vi "Parse Diff Report to Text.vi"(0 "XML Path":path, 1 "Ignore cosmetic changes? (T)":bool=TRUE, 2 "Attributes only? (F)":bool, 11 "error in":errorcluster) -> (4 "change description":string, 15 "error out":errorcluster)   [LabVIEW 2020, in "Graphical Diff.lvlib"]
uses:
  Graphical Diff.lvlib
  <vilib>/xml/NI_XML.lvlib
  <resource>/objmgr/DOMUserDefRef.rc
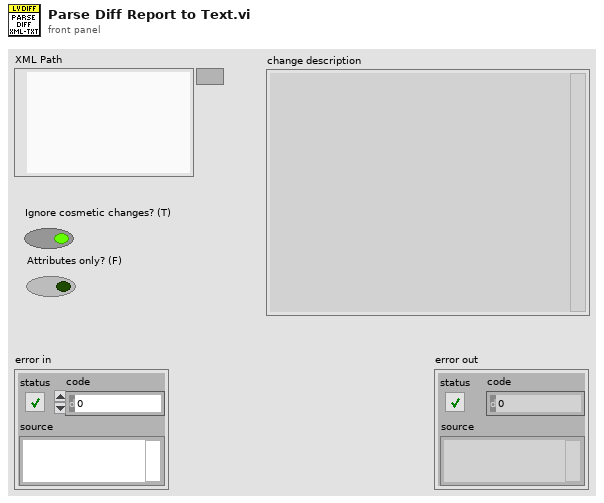
[diagram p1: front panel]
types:
  T1 = cluster{"Value":string, "Value":string, "Value":string, "Value":string}
  T2 = cluster{"Value":string, "Value":string, "Value":string, "Value":string}[]
  T3 = cluster{string, cluster{"Value":string, "Value":string, "Value":string, "Value":string}[]}
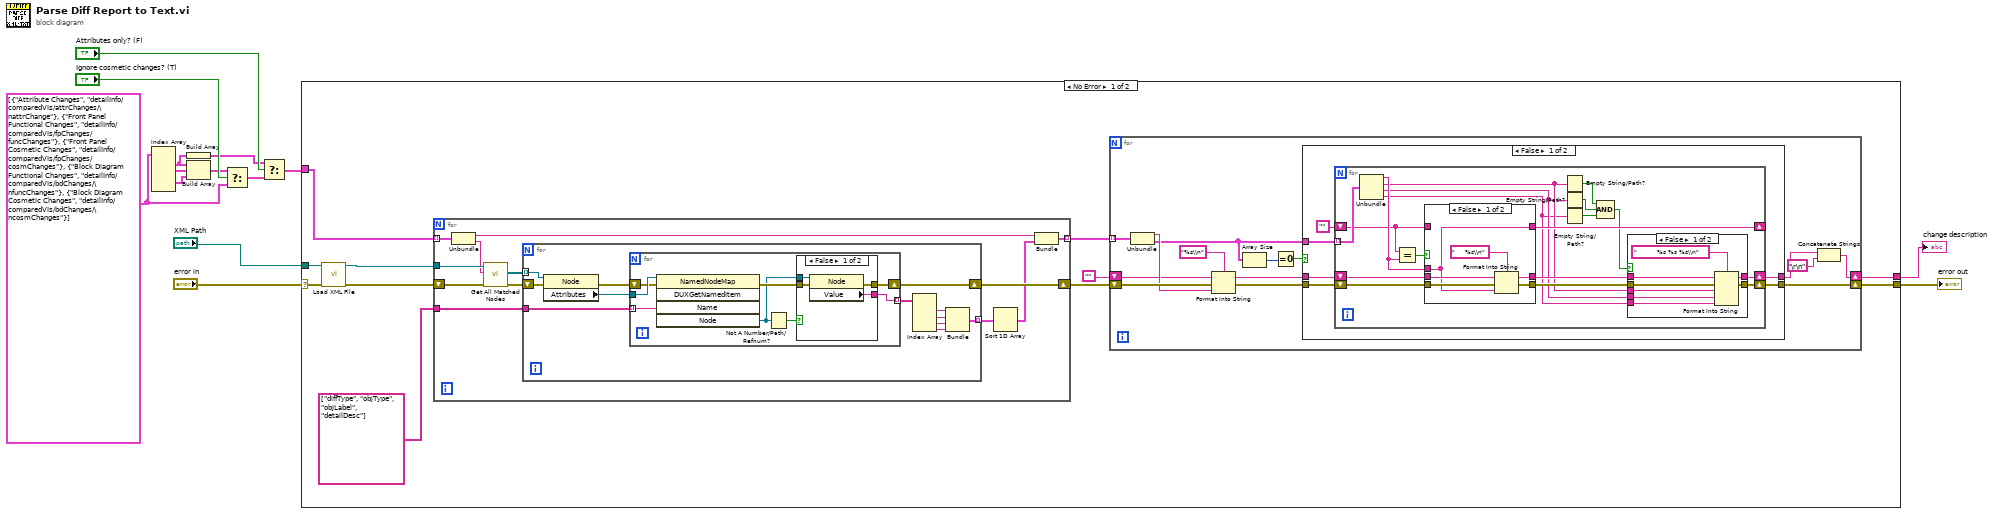
[diagram p0: block diagram]
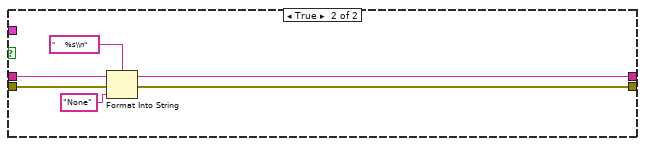
[diagram p4: hidden frame]
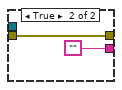
[diagram p5: hidden frame]
diagram:
  w5 = cluster{string, string}[] [{"Attribute Changes", "detailInfo/comparedVIs/attrChanges/\nattrChange"}, {"Front Panel Functional Changes", "detailInfo/comparedVIs/fpChanges/funcChanges"}, {"Front Panel Cosmetic Changes", "detailInfo/comparedVIs/fpChanges/cosmChanges"}, {"Block Diagram Functional Changes", "detailInfo/comparedVIs/bdChanges/\nfuncChanges"}, {"Block Diagram Cosmetic Changes", "detailInfo/comparedVIs/bdChanges/\ncosmChanges"}]
  n1 = Index Array(array=w5) -> (element #1=w8:cluster{string, string}, element #2=w9:cluster{string, string}, element #4=w10:cluster{string, string})  [unwired: 5 in, 2 out]
  n2 = Build Array(w8) -> (w3:cluster{string, string}[])
  n3 = Build Array(w8, w9, w10) -> (w6:cluster{string, string}[])
  n4 = Select(t=w6, s="Ignore cosmetic changes? (T)", f=w5) -> (s? t:f=w1:cluster{string, string}[])
  n5 = Select(t=w3, s="Attributes only? (F)", f=w1) -> (s? t:f=w2:cluster{string, string}[])
  n6 = case shown="No Error" "error in" {
    selector: "error in" -> [w25 w127]
    tunnel: "XML Path" -> [w24 _]
    tunnel: [w22 w127] -> w12
    tunnel: [w21 _] -> w11
    tunnel: w2 -> [w15 _]
    frame No Error {
      n7 = call <vilib>:"Load XML File.vi"("path to XML document"=w24, "error in (no error)"=w25) -> ("DOM document out"=w20:refnum<k20>, "error out"=w19:errorcluster)  [unwired: 11 in, 1 out]
      n8 = for {
        tunnel: w20 -> [w100]
        shift-right: [w97] -> w16
        shift-left: w19 -> [w99]
        tunnel: w15 -> [w94] mode=indexing
        tunnel: string[] ["diffType", "objType", "objLabel", "detailDesc"] -> [w96]
        tunnel: [w89] -> w18 mode=indexing
        n9 = Unbundle(w94) -> (w90:string, w93:string)
        n10 = call <vilib>:"Get All Matched Nodes.vi"("error in (no error)"=w99, "XPath expression"=w93, "node in"=w100) -> ("error out"=w98:errorcluster, "node result array"=w92:refnum<k20>[])  [unwired: 6 in, 1 out]
        n11 = for {
          shift-right: [w109] -> w97
          shift-left: w98 -> [w110]
          tunnel: w96 -> [w108]
          tunnel: [w102] -> w95 mode=indexing
          tunnel: w92 -> [w101] mode=indexing
          n12 = property class="Node"(reference=w101, error in=w110) -> (error out=w112:errorcluster, "Attributes"=w111:refnum<k20>)  [unwired: 1 out]
          n13 = for {
            tunnel: w111 -> [w120]
            shift-right: [w116] -> w109
            shift-left: w112 -> [w119]
            tunnel: w108 -> [w118] mode=indexing
            tunnel: [w115] -> w107 mode=indexing
            n14 = invoke class="NamedNodeMap" method="DUXGetNamedItem"(reference=w120, error in=w119, "Name"=w118) -> (error out=w117:errorcluster, "Node"=w113:refnum<k20>)  [unwired: 2 in, 3 out]
            n15 = Not A Number/Path/Refnum?(number/path/refnum=w113) -> (NaN/Path/Refnum?=w114:bool)
            n16 = case shown="False" w114 {
              tunnel: w117 -> [w124 w126]
              tunnel: [w123 w126] -> w116
              tunnel: [w122 ""] -> w115
              tunnel: w113 -> [w121 _]
              frame False {
                n17 = property class="Node"(reference=w121, error in=w124) -> (error out=w123:errorcluster, "Value"=w122:string)  [unwired: 1 out]
              }
              frame True {
              }
            }
          }
          n18 = Index Array(array=w107) -> (element #1=w103:string, element #2=w106:string, element #3=w104:string, element #4=w105:string)  [unwired: 4 in]
          n19 = Bundle("Value"=w103, "Value"=w106, "Value"=w104, "Value"=w105) -> (w102:T1)  [unwired: 1 in]
        }
        n20 = Sort 1D Array(array=w95) -> (sorted array=w91:T2)
        n21 = Bundle(w90, w91) -> (w89:T3)  [unwired: 1 in]
      }
      n22 = for {
        tunnel: w18 -> [w39] mode=indexing
        shift-right: [w30] -> w22
        shift-left: w16 -> [w38]
        shift-right: [w27] -> w21
        shift-left: "" -> [w31]
        n23 = Unbundle(w39) -> (w37:string, w29:T2)
        n24 = Format Into String(format string="%s\\n", initial string=w31, error in=w38, w37) -> (resulting string=w32:string, error out=w33:errorcluster)
        n25 = Array Size(array=w29) -> (size(s)=w35:i32)
        n26 = Equal To 0?(x=w35) -> (x = 0?=w34:bool)
        n27 = case shown="False" w34 {
          tunnel: w33 -> [w45 w86]
          tunnel: w32 -> [w44 w85]
          tunnel: [w41 w84] -> w30
          tunnel: [w40 w83] -> w28
          tunnel: w29 -> [w43 _]
          frame False {
            n28 = for {
              shift-right: [w55] -> w41
              shift-left: w45 -> [w61]
              shift-right: [w54] -> w40
              shift-left: w44 -> [w60]
              tunnel: w43 -> [w63] mode=indexing
              shift-right: [w59] -> _
              shift-left: "" -> [w57]
              n29 = Unbundle(w63) -> ("Value"=w58:string, "Value"=w52:string, "Value"=w51:string, "Value"=w50:string)
              n30 = Equal?(x=w57, y=w58) -> (x = y?=w62:bool)
              n31 = case shown="False" w62 {
                tunnel: w61 -> [w78 w82]
                tunnel: w58 -> [w74 _]
                tunnel: w60 -> [w79 w81]
                tunnel: [w76 w82] -> w56
                tunnel: [w75 w81] -> w53
                tunnel: w57 -> [_ w80]
                tunnel: [w74 w80] -> w59
                frame False {
                  n32 = Format Into String(format string="     %s\\n", initial string=w79, error in=w78, w74) -> (resulting string=w75:string, error out=w76:errorcluster)
                }
                frame True {
                }
              }
              n33 = Empty String/Path?(string/path=w52) -> (empty?=w47:bool)
              n34 = Empty String/Path?(string/path=w51) -> (empty?=w48:bool)
              n35 = Empty String/Path?(string/path=w50) -> (empty?=w49:bool)
              n36 = Compound Arithmetic op=AND(w47, w48, w49) -> (w46:bool)
              n37 = case shown="False" w46 {
                tunnel: w56 -> [w71 w72]
                tunnel: [w70 w72] -> w55
                tunnel: [w68 w73] -> w54
                tunnel: w53 -> [w67 w73]
                tunnel: w52 -> [w66 _]
                tunnel: w51 -> [w65 _]
                tunnel: w50 -> [w64 _]
                frame False {
                  n38 = Format Into String(format string="          %s %s %s\\n", initial string=w67, error in=w71, w66, w65, w64) -> (resulting string=w68:string, error out=w70:errorcluster)
                }
                frame True {
                }
              }
            }
          }
          frame True {
            n39 = Format Into String(format string="     %s\\n", initial string=w85, error in=w86, "None" ("input 1")) -> (resulting string=w83:string, error out=w84:errorcluster)
          }
        }
        n40 = Concatenate Strings(w28, "\r\n") -> (w27:string)
      }
    }
    frame Error {
    }
  }
  "error out" <- w12
  "change description" <- w11
